vi "programa.vi"() -> ()   [LabVIEW 2020]
uses:
  Pos_def.vi
  Pos_Modf.vi
  vis_variables.vi
  Animaciones.vi
  Alarmas.vi
  Panela_R.vi
  Cuadrada.vi
panel:
  out "Pos Moldes_R 2":i32
  out "Pos Moldes_R":i32
  in  "Alarma Fuera de Norma":bool
  in  "Valvula de Filtro 3":bool
  in  "Alarma Baja Temperatura":bool
  in  "Alarma Alta Temperatura":bool
  in  "Alarma de llenado":bool
  in  "Valvula de Filtro":bool
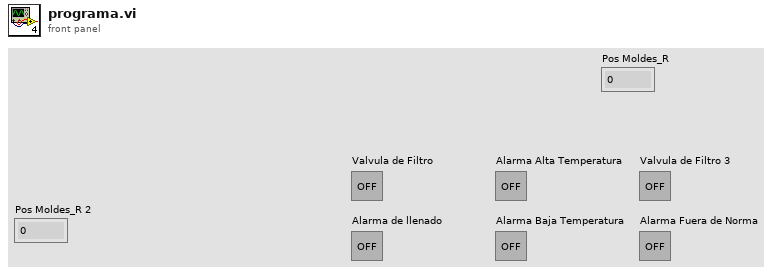
[diagram p1: front panel]
types:
  T1 = enum16{"Default", "Mover Camión", "Descargar Camión", "Mover Porcion Caña", "Filtrar", "Calentar", "Enfriar y Calentar"}
  T2 = enum16{"Default", "Mover Camión", "Descargar Camión"}
  T3 = enum16{"Default", "Mover Camión", "Descargar Camión", "Mover Porcion Caña", "Filtrar"}
  T4 = enum16{"Default", "Mover Camión", "Descargar Camión", "Mover Porcion Caña"}
  T5 = enum16{"Default", "Mover Camión", "Descargar Camión", "Mover Porcion Caña", "Filtrar", "Calentar"}
  T6 = cluster{"Pos Carro Caña":i32, "Pos Porcion Caña ":i32, "Pos Moldes_R":i32, "Pos Panelas_R":i32, "Pos Panelas_C":i32, "Pos Moldes _C":i32}
  T7 = cluster{"Pos_Modf_Carro_Caña":i32, "Pos_Modf_Porcion_Caña":i32, "Pos_Modf_Molde_Redondo":i32, "Pos_Modf_Molde_Cuadrado":i32, "Pos_Modf_Panela_R":i32, "Pos_Modf_Panela_C":i32}
  T8 = cluster{"vis carro caña":bool, "vis carro  vaciando":bool, "vis caña":bool, "vis porcion de caña":bool, "vis bagazo":bool, "vis guarapo":bool, " vis panela liquida":bool, " vis molde redondo":bool, " vis molde cuadrado":bool}
  T9 = cluster{"A_llenado":bool, "A_T_Fuera_Norma":bool, "A_Alta_temperatura":bool, "A_Baja_temperatura ":bool}
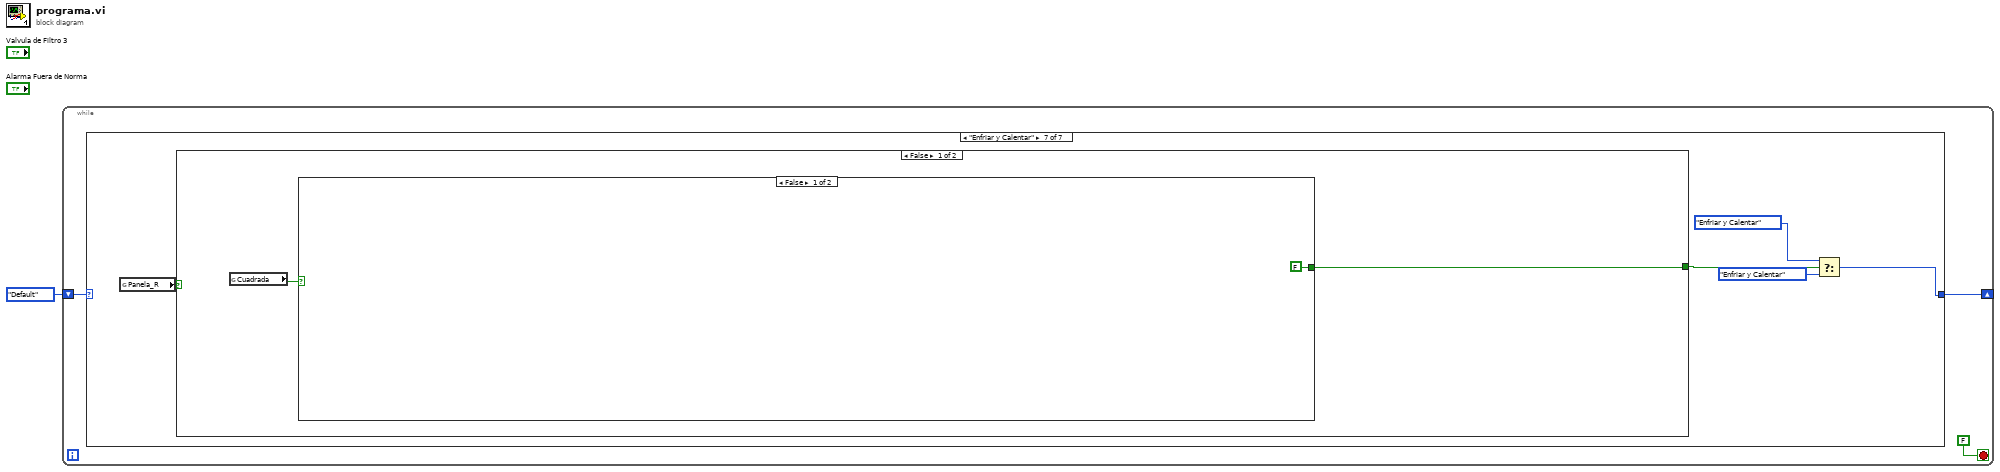
[diagram p0: block diagram]
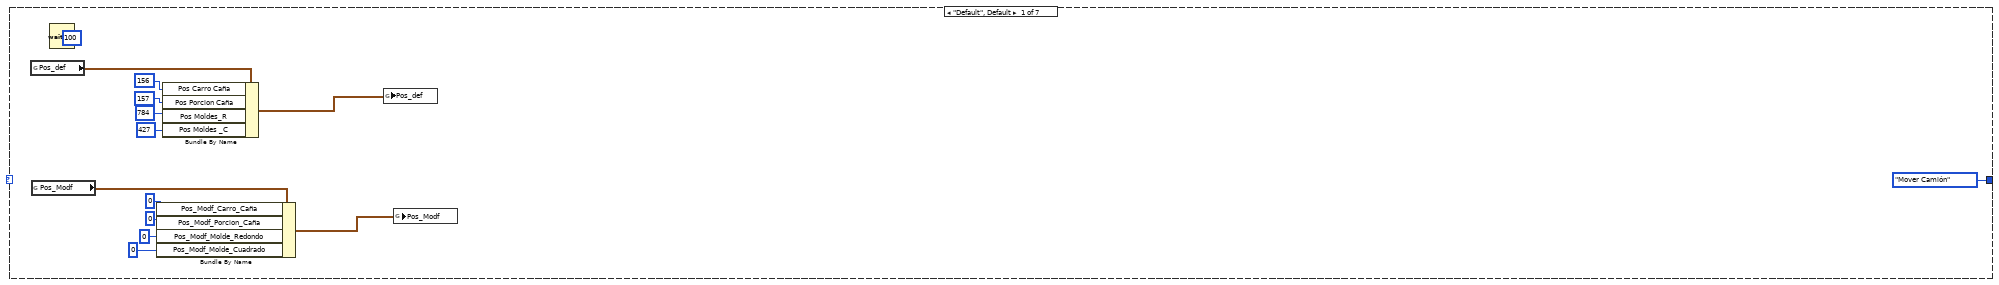
[diagram p2: hidden frame]
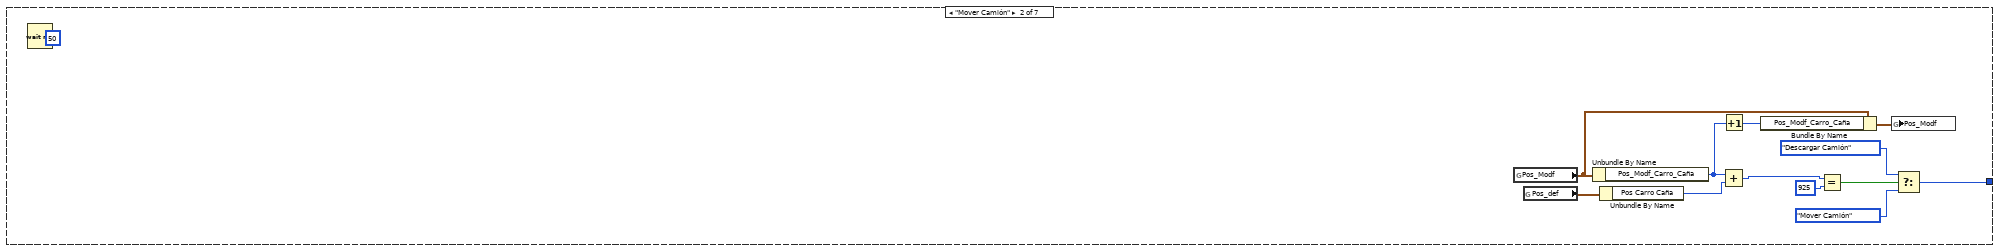
[diagram p3: hidden frame]
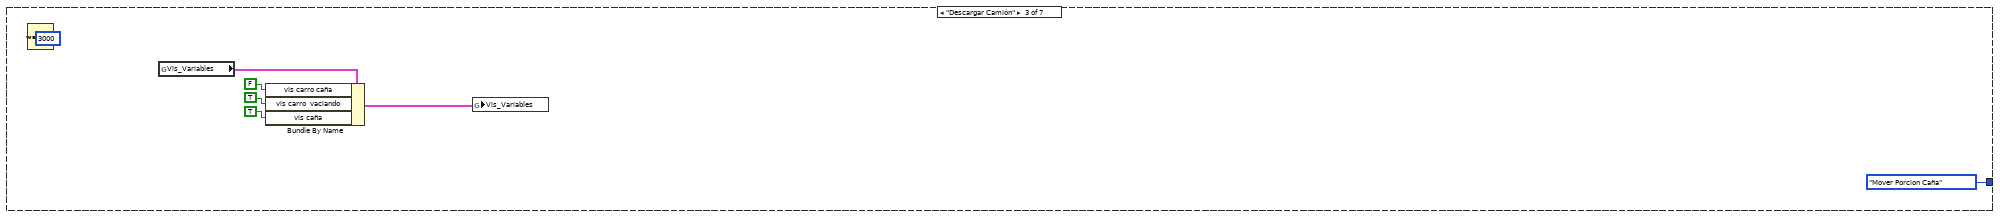
[diagram p4: hidden frame]
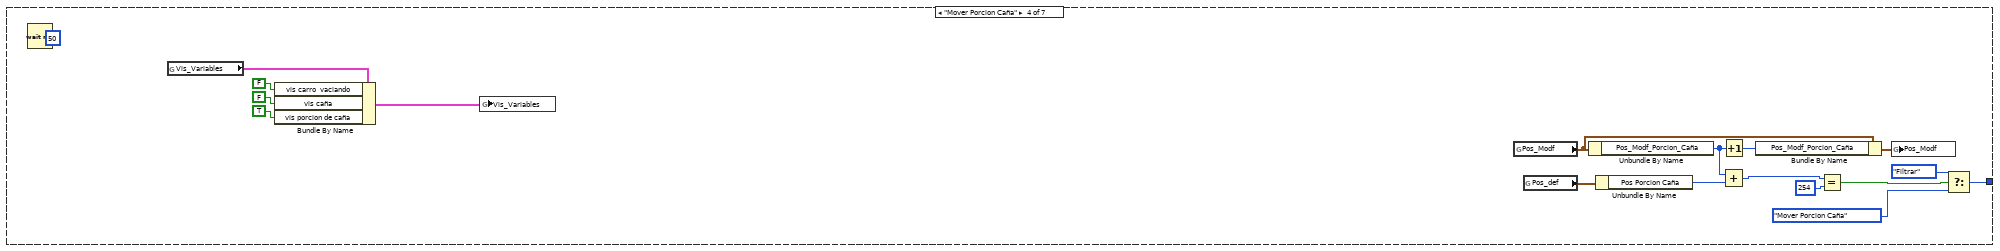
[diagram p5: hidden frame]
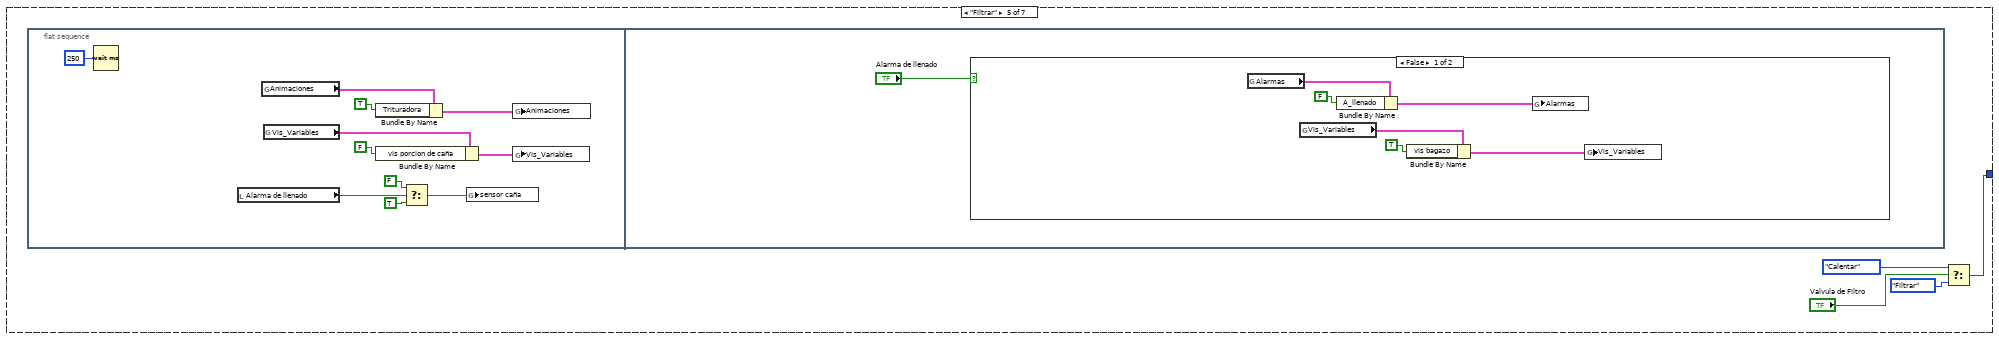
[diagram p6: hidden frame]
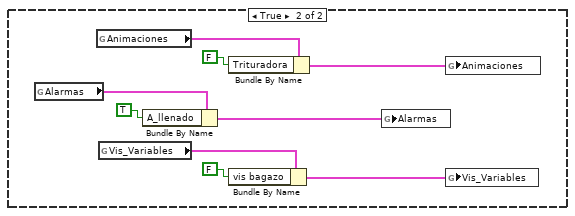
[diagram p7: hidden frame]
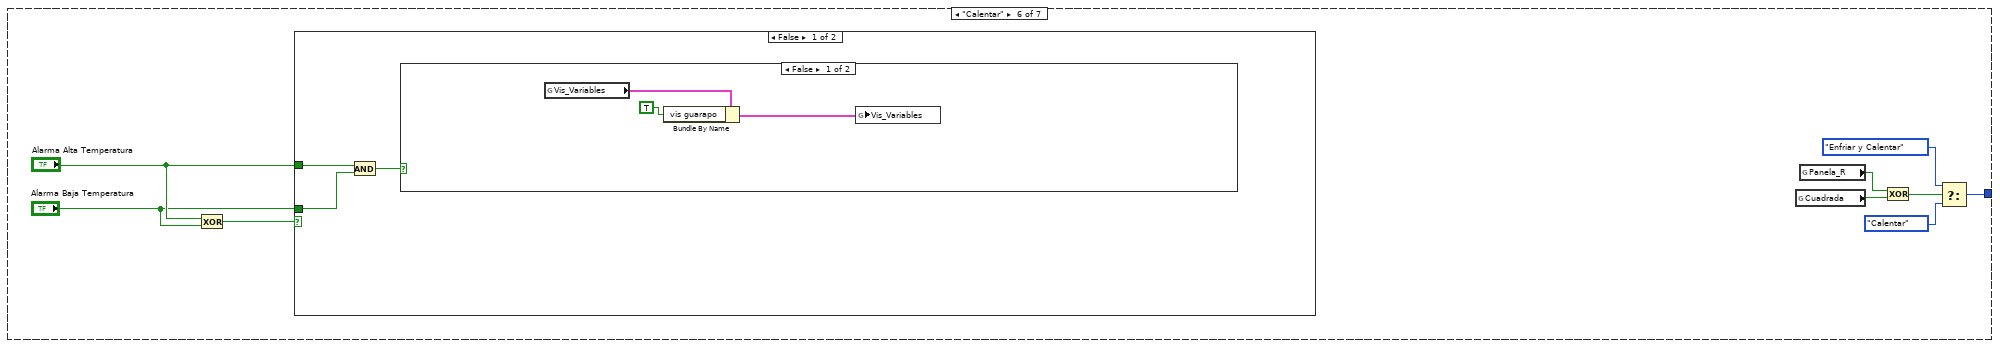
[diagram p8: hidden frame]
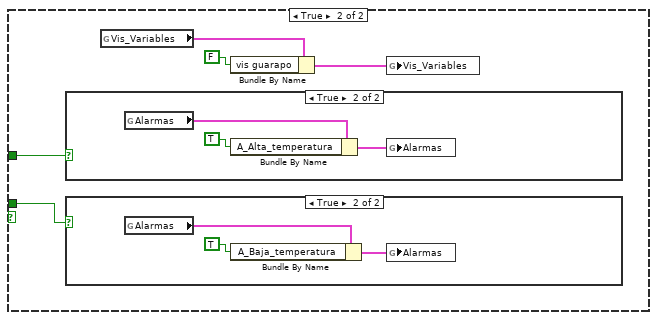
[diagram p10: hidden frame]
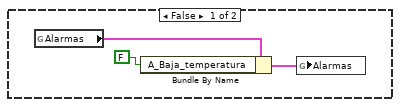
[diagram p11: hidden frame]
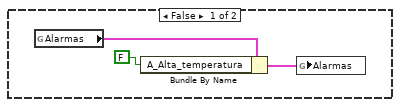
[diagram p12: hidden frame]
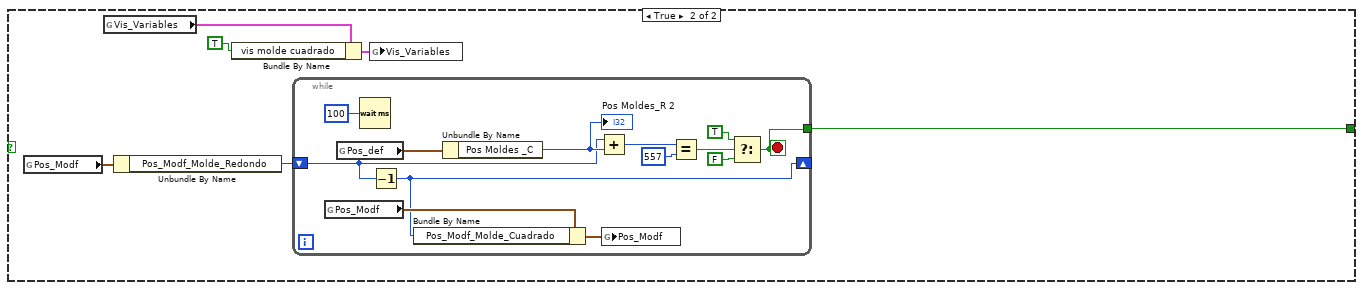
[diagram p13: hidden frame]
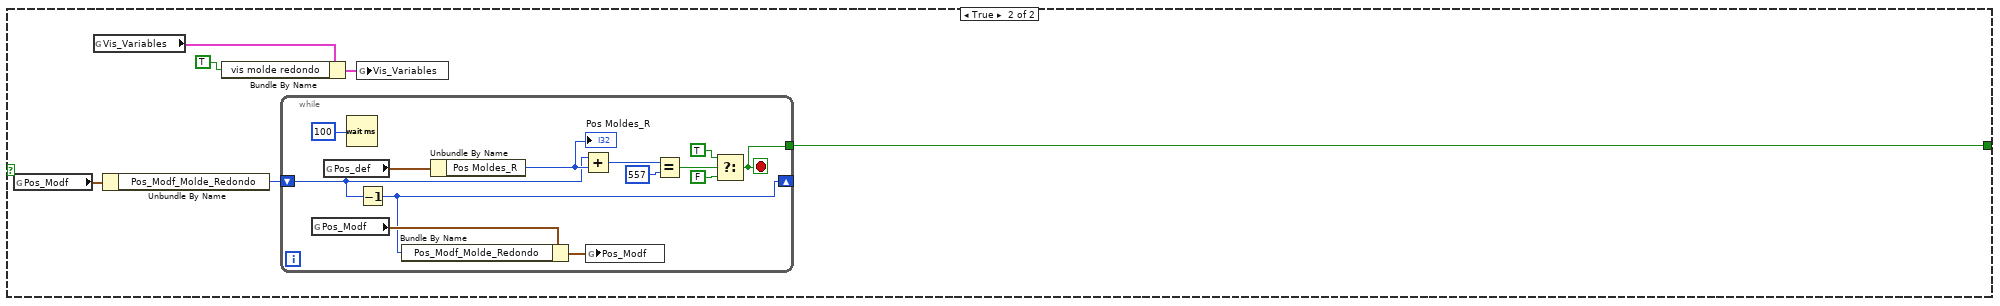
[diagram p14: hidden frame]
diagram:
  n1 = while {
    shift-right: [w2] -> _
    shift-left: T1."Default" -> [w3]
    stop <- FALSE stop-if-true
    n2 = case shown="\"Enfriar y Calentar\"" w3 {
      tunnel: [T2."Mover Camión" w24 T4."Mover Porcion Caña" w39 w57 w88 w120] -> w2
      frame "Default", Default {
        n3 = global read "Pos_def.vi" "Pos_def"() -> (w14:T6)
        n4 = global read "Pos_Modf.vi" "Pos_Modf"() -> (w16:T7)
        n5 = Wait (ms)(milliseconds to wait=u32 100) -> ()  [unwired: 1 out]
        n6 = Bundle By Name(cluster=w16, "Pos_Modf_Carro_Caña"=0, "Pos_Modf_Porcion_Caña"=0, "Pos_Modf_Molde_Redondo"=0, "Pos_Modf_Molde_Cuadrado"=0) -> (w15:T7)
        n7 = Bundle By Name(cluster=w14, "Pos Carro Caña"=156, "Pos Porcion Caña"=157, "Pos Moldes_R"=784, "Pos Moldes _C"=427) -> (w13:T6)
        n8 = global write "Pos_def.vi" "Pos_def"(w13) -> ()
        n9 = global write "Pos_Modf.vi" "Pos_Modf"(w15) -> ()
      }
      frame "Mover Camión" {
        n10 = Wait (ms)(milliseconds to wait=u32 50) -> ()  [unwired: 1 out]
        n11 = global read "Pos_Modf.vi" "Pos_Modf"() -> (w31:T7)
        n12 = global read "Pos_def.vi" "Pos_def"() -> (w29:T6)
        n13 = Unbundle By Name(w31) -> ("Pos_Modf_Carro_Caña"=w22:i32)
        n14 = Unbundle By Name(w29) -> ("Pos Carro Caña"=w28:i32)
        n15 = Add(x=w22, y=w28) -> (x+y=w27:i32)
        n16 = Increment(x=w22) -> (x+1=w21:i32)
        n17 = Bundle By Name(cluster=w31, "Pos_Modf_Carro_Caña"=w21) -> (w30:T7)
        n18 = Equal?(x=w27, y=925) -> (x = y?=w25:bool)
        n19 = global write "Pos_Modf.vi" "Pos_Modf"(w30) -> ()
        n20 = Select(t=T3."Descargar Camión", s=w25, f=T3."Mover Camión") -> (s? t:f=w24:T3)
      }
      frame "Descargar Camión" {
        n21 = Wait (ms)(milliseconds to wait=u32 3000) -> ()  [unwired: 1 out]
        n22 = global read "vis_variables.vi" "Vis_Variables"() -> (w38:T8)
        n23 = Bundle By Name(cluster=w38, "vis carro caña"=FALSE, "vis carro  vaciando"=TRUE, "vis caña"=TRUE) -> (w35:T8)
        n24 = global write "vis_variables.vi" "Vis_Variables"(w35) -> ()
      }
      frame "Mover Porcion Caña" {
        n25 = Wait (ms)(milliseconds to wait=u32 50) -> ()  [unwired: 1 out]
        n26 = global read "vis_variables.vi" "Vis_Variables"() -> (w52:T8)
        n27 = Bundle By Name(cluster=w52, "vis carro  vaciando"=FALSE, "vis caña"=FALSE, "vis porcion de caña"=TRUE) -> (w50:T8)
        n28 = global write "vis_variables.vi" "Vis_Variables"(w50) -> ()
        n29 = global read "Pos_Modf.vi" "Pos_Modf"() -> (w56:T7)
        n30 = global read "Pos_def.vi" "Pos_def"() -> (w47:T6)
        n31 = Unbundle By Name(w56) -> ("Pos_Modf_Porcion_Caña"=w46:i32)
        n32 = Unbundle By Name(w47) -> ("Pos Porcion Caña"=w45:i32)
        n33 = Add(x=w46, y=w45) -> (x+y=w44:i32)
        n34 = Increment(x=w46) -> (x+1=w55:i32)
        n35 = Bundle By Name(cluster=w56, "Pos_Modf_Porcion_Caña"=w55) -> (w54:T7)
        n36 = Equal?(x=w44, y=254) -> (x = y?=w42:bool)
        n37 = global write "Pos_Modf.vi" "Pos_Modf"(w54) -> ()
        n38 = Select(t=T3."Filtrar", s=w42, f=T3."Mover Porcion Caña") -> (s? t:f=w39:T3)
      }
      frame "Filtrar" {
        n39 = flat-sequence {
          frame #0 {
            n40 = Wait (ms)(milliseconds to wait=u32 250) -> ()  [unwired: 1 out]
            n41 = local read "Alarma de llenado"() -> (w61:bool)
            n42 = global read "Animaciones.vi" "Animaciones"() -> (w68:cluster{"Trituradora":bool, " Caja":bool})
            n43 = global read "vis_variables.vi" "Vis_Variables"() -> (w71:T8)
            n44 = Bundle By Name(cluster=w68, "Trituradora"=TRUE) -> (w66:cluster{"Trituradora":bool, " Caja":bool})
            n45 = Bundle By Name(cluster=w71, "vis porcion de caña"=FALSE) -> (w70:T8)
            n46 = Select(t=FALSE, s=w61, f=TRUE) -> (s? t:f=w62:bool)
            n47 = global write "senor caña.vi" "sensor caña"(w62) -> ()
            n48 = global write "Animaciones.vi" "Animaciones"(w66) -> ()
            n49 = global write "vis_variables.vi" "Vis_Variables"(w70) -> ()
          }
          frame #1 {
            n50 = case shown="False" "Alarma de llenado" {
              frame False {
                n51 = global read "Alarmas.vi" "Alarmas"() -> (w77:T9)
                n52 = global read "vis_variables.vi" "Vis_Variables"() -> (w76:T8)
                n53 = Bundle By Name(cluster=w77, "A_llenado"=FALSE) -> (w78:T9)
                n54 = Bundle By Name(cluster=w76, "vis bagazo"=TRUE) -> (w75:T8)
                n55 = global write "Alarmas.vi" "Alarmas"(w78) -> ()
                n56 = global write "vis_variables.vi" "Vis_Variables"(w75) -> ()
              }
              frame True {
                n57 = global read "Alarmas.vi" "Alarmas"() -> (w84:T9)
                n58 = global read "Animaciones.vi" "Animaciones"() -> (w81:cluster{"Trituradora":bool, " Caja":bool})
                n59 = global read "vis_variables.vi" "Vis_Variables"() -> (w85:T8)
                n60 = Bundle By Name(cluster=w84, "A_llenado"=TRUE) -> (w82:T9)
                n61 = Bundle By Name(cluster=w81, "Trituradora"=FALSE) -> (w79:cluster{"Trituradora":bool, " Caja":bool})
                n62 = Bundle By Name(cluster=w85, "vis bagazo"=FALSE) -> (w87:T8)
                n63 = global write "Alarmas.vi" "Alarmas"(w82) -> ()
                n64 = global write "Animaciones.vi" "Animaciones"(w79) -> ()
                n65 = global write "vis_variables.vi" "Vis_Variables"(w87) -> ()
              }
            }
          }
        }
        n66 = Select(t=T5."Calentar", s="Valvula de Filtro", f=T5."Filtrar") -> (s? t:f=w57:T5)
      }
      frame "Calentar" {
        n67 = Exclusive Or(1:"Alarma Baja Temperatura", 2:"Alarma Alta Temperatura") -> (0:w96:bool)
        n68 = case shown="False" w96 {
          tunnel: "Alarma Alta Temperatura" -> [w99 w104]
          tunnel: "Alarma Baja Temperatura" -> [w98 w103]
          frame False {
            n69 = And(x=w99, y=w98) -> (x .and. y?=w97:bool)
            n70 = case shown="False" w97 {
              frame False {
                n71 = global read "vis_variables.vi" "Vis_Variables"() -> (w101:T8)
                n72 = Bundle By Name(cluster=w101, "vis guarapo"=TRUE ("vis bagazo")) -> (w102:T8)
                n73 = global write "vis_variables.vi" "Vis_Variables"(w102) -> ()
              }
              frame True {
              }
            }
          }
          frame True {
            n74 = case shown="True" w104 {
              frame False {
                n75 = global read "Alarmas.vi" "Alarmas"() -> (w114:T9)
                n76 = Bundle By Name(cluster=w114, "A_Alta_temperatura"=FALSE) -> (w116:T9)
                n77 = global write "Alarmas.vi" "Alarmas"(w116) -> ()
              }
              frame True {
                n78 = global read "Alarmas.vi" "Alarmas"() -> (w119:T9)
                n79 = Bundle By Name(cluster=w119, "A_Alta_temperatura"=TRUE) -> (w118:T9)
                n80 = global write "Alarmas.vi" "Alarmas"(w118) -> ()
              }
            }
            n81 = case shown="True" w103 {
              frame False {
                n82 = global read "Alarmas.vi" "Alarmas"() -> (w110:T9)
                n83 = Bundle By Name(cluster=w110, "A_Baja_temperatura"=FALSE ("A_Alta_temperatura")) -> (w108:T9)
                n84 = global write "Alarmas.vi" "Alarmas"(w108) -> ()
              }
              frame True {
                n85 = global read "Alarmas.vi" "Alarmas"() -> (w113:T9)
                n86 = Bundle By Name(cluster=w113, "A_Baja_temperatura"=TRUE ("A_Alta_temperatura")) -> (w111:T9)
                n87 = global write "Alarmas.vi" "Alarmas"(w111) -> ()
              }
            }
            n88 = global read "vis_variables.vi" "Vis_Variables"() -> (w107:T8)
            n89 = Bundle By Name(cluster=w107, "vis guarapo"=FALSE ("vis bagazo")) -> (w106:T8)
            n90 = global write "vis_variables.vi" "Vis_Variables"(w106) -> ()
          }
        }
        n91 = global read "Cuadrada.vi" "Cuadrada"() -> (w92:bool)
        n92 = global read "Panela_R.vi" "Panela_R"() -> (w93:bool)
        n93 = Exclusive Or(1:w92, 2:w93) -> (0:w91:bool)
        n94 = Select(t=T1."Enfriar y Calentar", s=w91, f=T1."Calentar") -> (s? t:f=w88:T1)
      }
      frame "Enfriar y Calentar" {
        n95 = global read "Panela_R.vi" "Panela_R"() -> (w124:bool)
        n96 = case shown="False" w124 {
          tunnel: [w125 w147] -> w123
          frame False {
            n97 = global read "Cuadrada.vi" "Cuadrada"() -> (w126:bool)
            n98 = case shown="False" w126 {
              tunnel: [FALSE ("t") w128] -> w125
              frame False {
              }
              frame True {
                n99 = global read "Pos_Modf.vi" "Pos_Modf"() -> (w130:T7)
                n100 = global read "vis_variables.vi" "Vis_Variables"() -> (w133:T8)
                n101 = Unbundle By Name(w130) -> ("Pos_Modf_Molde_Redondo"=w129:i32)
                n102 = Bundle By Name(cluster=w133, "vis molde cuadrado"=TRUE ("vis molde redondo")) -> (w131:T8)
                n103 = while {
                  shift-right: [w141] -> _
                  shift-left: w129 -> [w142]
                  tunnel: [w134] -> w128
                  stop <- w134 stop-if-true
                  n104 = global read "Pos_Modf.vi" "Pos_Modf"() -> (w145:T7)
                  n105 = global read "Pos_def.vi" "Pos_def"() -> (w146:T6)
                  n106 = Wait (ms)(milliseconds to wait=u32 100) -> ()  [unwired: 1 out]
                  n107 = Decrement(x=w142) -> (x-1=w141:i32)
                  n108 = Bundle By Name(cluster=w145, "Pos_Modf_Molde_Cuadrado"=w141) -> (w144:T7)
                  n109 = Unbundle By Name(w146) -> ("Pos Moldes _C"=w143:i32)
                  "Pos Moldes_R 2" <- w143
                  n110 = Add(x=w142, y=w143) -> (x+y=w140:i32)
                  n111 = global write "Pos_Modf.vi" "Pos_Modf"(w144) -> ()
                  n112 = Equal?(x=w140, y=557) -> (x = y?=w138:bool)
                  n113 = Select(t=TRUE, s=w138, f=FALSE) -> (s? t:f=w134:bool)
                }
                n114 = global write "vis_variables.vi" "Vis_Variables"(w131) -> ()
              }
            }
          }
          frame True {
            n115 = global read "Pos_Modf.vi" "Pos_Modf"() -> (w149:T7)
            n116 = global read "vis_variables.vi" "Vis_Variables"() -> (w152:T8)
            n117 = Unbundle By Name(w149) -> ("Pos_Modf_Molde_Redondo"=w148:i32)
            n118 = Bundle By Name(cluster=w152, "vis molde redondo"=TRUE) -> (w150:T8)
            n119 = while {
              shift-right: [w160] -> _
              shift-left: w148 -> [w161]
              tunnel: [w153] -> w147
              stop <- w153 stop-if-true
              n120 = global read "Pos_Modf.vi" "Pos_Modf"() -> (w164:T7)
              n121 = global read "Pos_def.vi" "Pos_def"() -> (w165:T6)
              n122 = Wait (ms)(milliseconds to wait=u32 100) -> ()  [unwired: 1 out]
              n123 = Decrement(x=w161) -> (x-1=w160:i32)
              n124 = Bundle By Name(cluster=w164, "Pos_Modf_Molde_Redondo"=w160) -> (w163:T7)
              n125 = Unbundle By Name(w165) -> ("Pos Moldes_R"=w162:i32)
              "Pos Moldes_R" <- w162
              n126 = Add(x=w161, y=w162) -> (x+y=w159:i32)
              n127 = global write "Pos_Modf.vi" "Pos_Modf"(w163) -> ()
              n128 = Equal?(x=w159, y=557) -> (x = y?=w157:bool)
              n129 = Select(t=TRUE, s=w157, f=FALSE) -> (s? t:f=w153:bool)
            }
            n130 = global write "vis_variables.vi" "Vis_Variables"(w150) -> ()
          }
        }
        n131 = Select(t=T1."Enfriar y Calentar", s=w123, f=T1."Enfriar y Calentar") -> (s? t:f=w120:T1)
      }
    }
  }
